vi "GetVersionSerializableData.vi"(10 "Version":u16, 11 "DNL_LabVIEW Object in":refnum<class "BlueSerializableTemplate.lvclass">) -> (0 "error out":errorcluster, 1 "Found?":bool, 2 "SerializableData":variant, 3 "DNL_LabVIEW Object out":refnum<class "BlueSerializableTemplate.lvclass">)   [LabVIEW 2019, in "BlueSerializableTemplate.lvlib" / "BlueSerializableTemplate.lvclass"]
uses:
  BlueSerializableTemplate.lvclass
  SerializableData.ctl
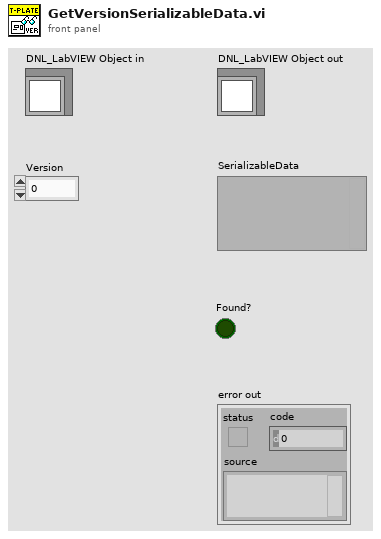
[diagram p1: front panel]
types:
  T1 = typedef "BlueSerializableTemplate.lvlib/BlueSerializableTemplate.lvclass/SerializableData.ctl" = cluster{"Placeholder":bool}
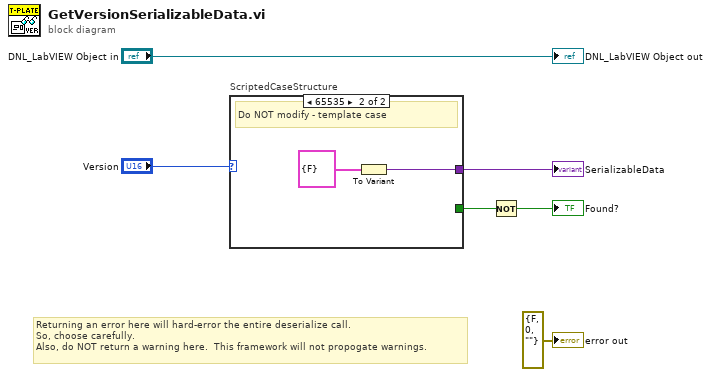
[diagram p0: block diagram]
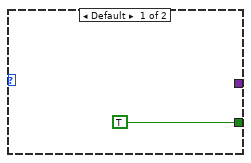
[diagram p2: hidden frame]
diagram:
  # "Returning an error here will hard-error the entire deserialize call.\nSo, choose carefully.\nAlso, do NOT return a warning here.  This framework will not propogate warnings."
  n1 = case "ScriptedCaseStructure" shown="65535" "Version" {
    tunnel: [_ w9] -> w5
    tunnel: [TRUE _] -> w4
    frame Default {
    }
    frame 65535 {
      # "Do NOT modify - template case"
      n2 = To Variant(anything=T1 {"Placeholder"=FALSE} ("SerializableData")) -> (Variant=w9:variant)
    }
  }
  "SerializableData" <- w5
  n3 = Not(x=w4) -> (.not. x?=→"Found?":bool)
  "error out" <- errorcluster {"status"=FALSE, "code"=0, "source"=""} ("error out")
  "DNL_LabVIEW Object out" <- "DNL_LabVIEW Object in"
